vi "FestoCPX.Station.ButtonsLed.Set.vi"(8 "error in":errorcluster, 10 "Buttons.State (OFF)":T1) -> (0 "error out":errorcluster)   [LabVIEW 2016]
uses:
  FestoCPX.Station.ButtonsState.ctl
  FestoCPX.DO.Signal.ctl
  FestoCPX.Station.TowerLed.Fglb.Action.ctl
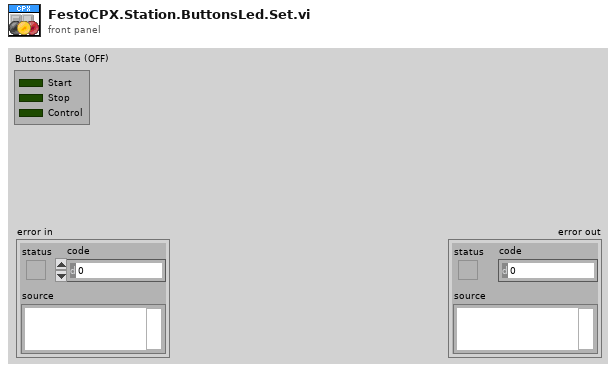
[diagram p1: front panel]
types:
  T1 = typedef "FestoCPX.Station.ButtonsState.ctl" = cluster{"Start":bool, "Stop":bool, "Control":bool}
  T2 = typedef "FestoCPX.Station.TowerLed.Fglb.Action.ctl" = enum16{"init", "set", "get"}
  T3 = typedef "FestoCPX.DO.Signal.ctl" = enum16{"Safety Reset", "Air Main Valve", "Door Lock", "Button LED Start", "Button LED Stop", "Button LED Control", "Traffic LED Red", "Traffic LED Orange", "Traffic LED Green", "Horn", "Laser Interlock", "Laser Trigger", "Laser Fume Extractor", "Product Suction Gripper Slot 1 A", "Product Suction Gripper Slot 1 B", "Product Suction Gripper Slot 2 A", "Product Suction Gripper Slot 2 B", "Product Suction Gripper Slot 3 A", "Product Suction Gripper Slot 3 B", "Product Suction Gripper Slot 4 A", "Product Suction Gripper Slot 4 B", "Product Suction Gripper Final A", "Product Suction Gripper Final B", "Lamp", "Q1 Product Move Work", "Q1 Product Move Home", "Q2 Table Turn Work", "Q2 Table Turn Home", "Q3 Product Lift A", "Q3 Product Lift B", "Q4 Product Arm OK", "Q4 Product Arm NOK", "Q5 Product Arm Work", "Q6 Product BlowOut A", "Q6 Product BlowOut B"}
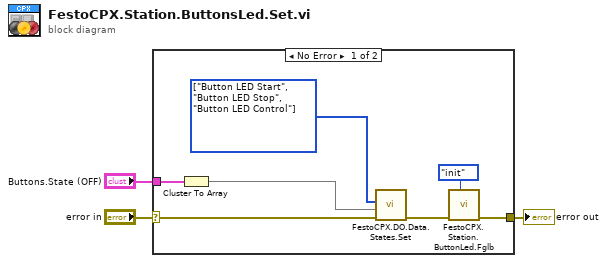
[diagram p0: block diagram]
diagram:
  n1 = case shown="No Error" "error in" {
    selector: "error in" -> [w10 w11]
    tunnel: [w4 w11] -> w3
    tunnel: "Buttons.State (OFF)" -> [w8 _]
    frame No Error {
      w9 = T3[] [enum."Button LED Start", enum."Button LED Stop", enum."Button LED Control"] items=["Safety Reset", "Air Main Valve", "Door Lock", "Button LED Start", "Button LED Stop", "Button LED Control", "Traffic LED Red", "Traffic LED Orange", "Traffic LED Green", "Horn", "Laser Interlock", "Laser Trigger", "Laser Fume Extractor", "Product Suction Gripper Slot 1 A", "Product Suction Gripper Slot 1 B", "Product Suction Gripper Slot 2 A", "Product Suction Gripper Slot 2 B", "Product Suction Gripper Slot 3 A", "Product Suction Gripper Slot 3 B", "Product Suction Gripper Slot 4 A", "Product Suction Gripper Slot 4 B", "Product Suction Gripper Final A", "Product Suction Gripper Final B", "Lamp", "Q1 Product Move Work", "Q1 Product Move Home", "Q2 Table Turn Work", "Q2 Table Turn Home", "Q3 Product Lift A", "Q3 Product Lift B", "Q4 Product Arm OK", "Q4 Product Arm NOK", "Q5 Product Arm Work", "Q6 Product BlowOut A", "Q6 Product BlowOut B"] ("CPX.DI")
      n2 = Cluster To Array(cluster=w8) -> (array=w7:bool[])
      n3 = call "FestoCPX.DO.Data.States.Set.vi"("error in (no error)"=w10, "State"=w7, "CPX.DO"=w9) -> ("error out"=w5:errorcluster)  [unwired: 8 in]
      n4 = call "FestoCPX.Station.ButtonLed.Fglb.vi"("Action (get)"=FestoCPX.Station.TowerLed.Fglb.Action."init", "error in"=w5) -> ("error out"=w4:errorcluster)  [unwired: 7 in, 2 out]
    }
    frame Error {
    }
  }
  "error out" <- w3
